vi "TRITON_RI_CLOSE.vi"(1 "error in (no error)":errorcluster, 2 "Communication Cluster":T1) -> (0 "error out":errorcluster)   [LabVIEW 2019]
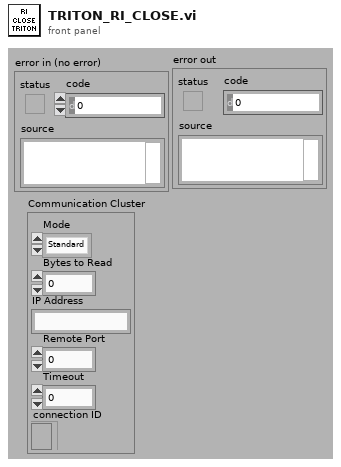
[diagram p1: front panel]
types:
  T1 = cluster{"Mode":enum16{"Standard", "Buffered", "CRLF", "Immediate"}, "Bytes to Read":i32, "IP Address":string, "Remote Port":i32, "Timeout":i32, "connection ID":refnum<k5>}
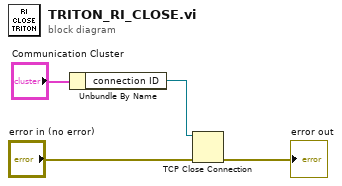
[diagram p0: block diagram]
diagram:
  n1 = Unbundle By Name("Communication Cluster") -> ("connection ID"=w2:refnum<k5>)
  n2 = TCP Close Connection(connection ID=w2, error in (no error)="error in (no error)") -> (error out=→"error out":errorcluster)  [unwired: 1 in, 1 out]
